vi "BundleAll.vi"(8 "error in (no error)":errorcluster, 10 "Game in\natualized":refnum<class "Game.lvclass">, 11 "Game in":refnum<class "Game.lvclass">) -> (0 "error out":errorcluster, 3 "Game out":refnum<class "Game.lvclass">)   [LabVIEW 2018, in "Game.lvclass"]
uses:
  Game.lvclass
  Game.lvclass/Game.ctl
  Read AllyRef.vi
  Read BallRef.vi
  Read EnemyRef.vi
  Read FieldRef.vi
  Read Referee.vi
  Read TimeRef.vi
  Write AllyRef.vi
  Write BallRef.vi
  Write EnemyRef.vi
  Write FieldRef.vi
  Write Referee.vi
  Write TimeRef.vi
  Ally_class/Ally.lvclass
  Ball_class/Ball.lvclass
  Enemy_class/Enemy.lvclass
  Field_class/Field.lvclass
  Referee_class/Referee.lvclass
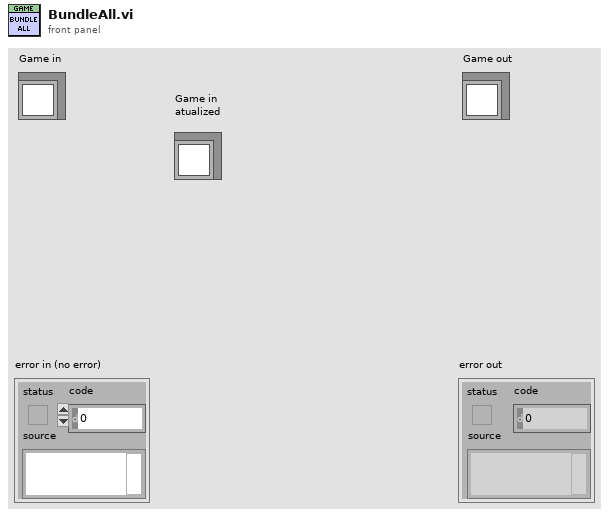
[diagram p1: front panel]
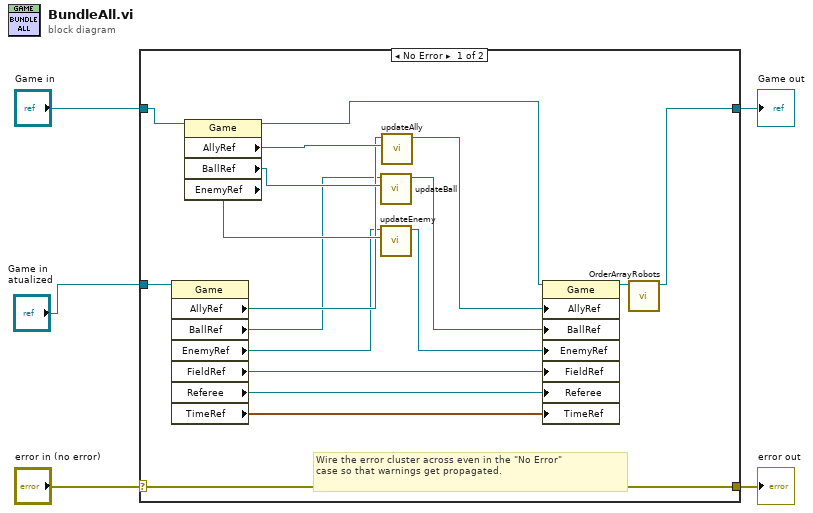
[diagram p0: block diagram]
diagram:
  n1 = case shown="No Error" "error in (no error)" {
    selector: "error in (no error)" -> [w23 w25]
    tunnel: [w23 w25] -> w4
    tunnel: [w8 w24] -> w2
    tunnel: "Game in" -> [w20 w24]
    tunnel: "Game in\natualized" -> [w22 _]
    frame No Error {
      # "Wire the error cluster across even in the \"No Error\"\ncase so that warnings get propagated."
      n2 = property class="Game"(reference=w22) -> ("AllyRef"=w16:refnum<class "Ally.lvclass">, "BallRef"=w15:refnum<class "Ball.lvclass">, "EnemyRef"=w14:refnum<class "Enemy.lvclass">, "FieldRef"=w7:refnum<class "Field.lvclass">, "Referee"=w6:refnum<class "Referee.lvclass">, "TimeRef"=w21:timestamp)  [unwired: 1 in, 2 out]
      n3 = property class="Game"(reference=w20) -> (reference out=w10:refnum<class "Game.lvclass">, "AllyRef"=w19:refnum<class "Ally.lvclass">, "BallRef"=w18:refnum<class "Ball.lvclass">, "EnemyRef"=w17:refnum<class "Enemy.lvclass">)  [unwired: 1 in, 1 out]
      n4 = call "updateBall.vi"("old Ball"=w18, "Ball in"=w15) -> ("Ball out"=w12:refnum<class "Ball.lvclass">)  [unwired: 8 in, 1 out]
      n5 = call "updateEnemy.vi"("old Enemy"=w17, "Enemy in"=w14) -> ("Enemy out"=w13:refnum<class "Enemy.lvclass">)  [unwired: 8 in, 1 out]
      n6 = call "updateAlly.vi"("Old Ally"=w19, "New Ally from Vision"=w16) -> ("Ally out"=w11:refnum<class "Ally.lvclass">)  [unwired: 8 in, 1 out]
      n7 = property class="Game"(reference=w10, "AllyRef"=w11, "BallRef"=w12, "EnemyRef"=w13, "FieldRef"=w7, "Referee"=w6, "TimeRef"=w21) -> (reference out=w9:refnum<class "Game.lvclass">)  [unwired: 1 in, 1 out]
      n8 = call-dynamic "OrderArrayRobots.vi"("Game in"=w9) -> ("Game out"=w8:refnum<class "Game.lvclass">)  [unwired: 9 in, 1 out]
    }
    frame Error {
    }
  }
  "error out" <- w4
  "Game out" <- w2
